vi "SpecAn OPC Complete.vi"(8 "Error In":errorcluster, 9 "Max Time (ms)":i32=10000, 11 "VISA In":refnum<visa-resource-name>) -> (0 "Error Out":errorcluster, 1 "TimedOut":bool, 2 "Completed":bool, 3 "VISA Out":refnum<visa-resource-name>, 5 "StatusByte":string)   [LabVIEW 2015]
uses:
  Controls/FGV Action SpecAn Model.ctl
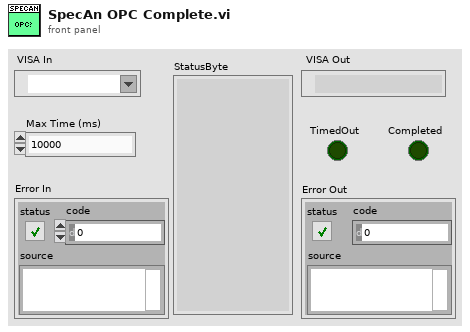
[diagram p1: front panel]
types:
  T1 = typedef "FGV Action SpecAn Model.ctl" = enum16{"Get", "Set"}
  T2 = typedef "SpecAn Model.ctl" = enum16{"E4440", "N9030"}
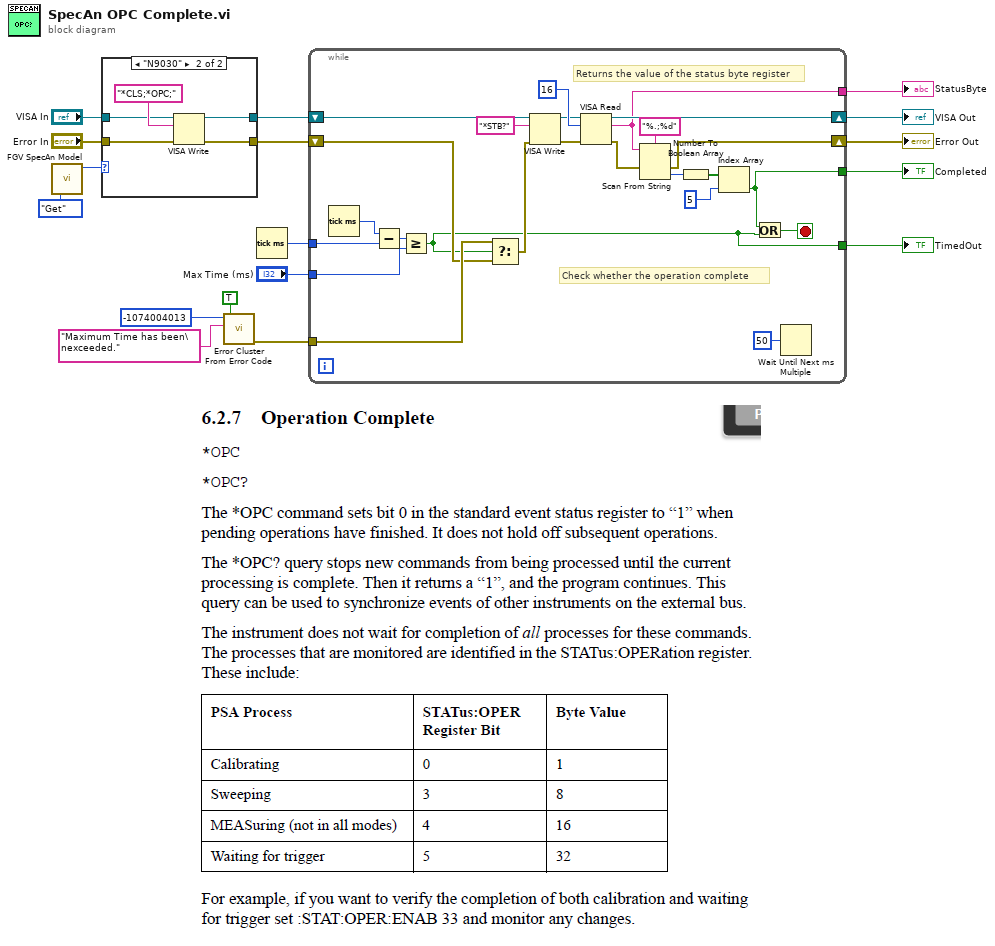
[diagram p0: block diagram]
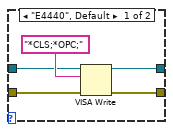
[diagram p2: hidden frame]
diagram:
  n1 = call "FGV SpecAn Model.vi"("Action"=FGV_Action_SpecAn_Model."Get") -> ("SA Model"=w1:T2)  [unwired: 6 in, 1 out]
  n2 = case shown="\"N9030\"" w1 {
    tunnel: [w22 w27] -> w11
    tunnel: [w21 w26] -> w10
    tunnel: "Error In" -> [w19 w24]
    tunnel: "VISA In" -> [w18 w23]
    frame "E4440", Default {
      n3 = VISA Write(VISA resource name=w18, write buffer="*CLS;*OPC;", error in (no error)=w19) -> (VISA resource name out=w22:refnum<visa-resource-name>, error out=w21:errorcluster)  [unwired: 1 out]
    }
    frame "N9030" {
      n4 = VISA Write(VISA resource name=w23, write buffer="*CLS;*OPC;", error in (no error)=w24) -> (VISA resource name out=w27:refnum<visa-resource-name>, error out=w26:errorcluster)  [unwired: 1 out]
    }
  }
  n5 = call <vilib>:"Error Cluster From Error Code.vi"("show call chain? (False)"=TRUE, "error message (\"\")"="Maximum Time has been\nexceeded." ("error message (\"\")"), "error code (0)"=-1074004013) -> ("error out"=w12:errorcluster)  [unwired: 6 in]
  n6 = Tick Count (ms)() -> (millisecond timer value=w16:u32)
  n7 = while {
    tunnel: "Max Time (ms)" -> [w34]
    tunnel: w16 -> [w43]
    tunnel: w12 -> [w31]
    shift-right: [w33] -> w9
    shift-left: w10 -> [w30]
    shift-right: [w50] -> w8
    shift-left: w11 -> [w47]
    tunnel: [w32] -> w7
    tunnel: [w29] -> w6
    tunnel: [w28] -> w5
    stop <- w38 stop-if-true
    # "Check whether the operation complete"
    # "Returns the value of the status byte register"
    n8 = Tick Count (ms)() -> (millisecond timer value=w44:u32)
    n9 = Subtract(x=w44, y=w43) -> (x-y=w35:u32)
    n10 = Greater Or Equal?(x=w35, y=w34) -> (x >= y?=w29:bool)
    n11 = Select(t=w31, s=w29, f=w30) -> (s? t:f=w37:errorcluster)
    n12 = VISA Write(VISA resource name=w47, write buffer="*STB?", error in (no error)=w37) -> (VISA resource name out=w45:refnum<visa-resource-name>, error out=w46:errorcluster)  [unwired: 1 out]
    n13 = VISA Read(VISA resource name=w45, byte count=u32 16, error in (no error)=w46) -> (VISA resource name out=w50:refnum<visa-resource-name>, read buffer=w28:string, error out=w42:errorcluster)  [unwired: 1 out]
    n14 = Scan From String(format string="%.;%d", input string=w28, error in=w42) -> (error out=w33:errorcluster, output 1=w39:i32)  [unwired: 2 in, 2 out]
    n15 = Number To Boolean Array(number=w39) -> (Boolean array=w40:bool[])
    n16 = Index Array(array=w40, index=5) -> (element=w32:bool)
    n17 = Or(x=w32, y=w29) -> (x .or. y?=w38:bool)
    n18 = Wait Until Next ms Multiple(millisecond multiple=u32 50 ("milliseconds to wait")) -> ()  [unwired: 1 out]
  }
  "Error Out" <- w9
  "VISA Out" <- w8
  "Completed" <- w7
  "TimedOut" <- w6
  "StatusByte" <- w5
